vi "begin_conveyor.vi"() -> (0 "error out":errorcluster)   [LabVIEW 2012]
uses:
  <vilib>/Rock Robotics/WPI/CAN/Jaguar/SubVIs/WPI_CANJaguar_BrakeCoastMode.ctl
  <vilib>/Rock Robotics/SystemInterfaces/AI/FPGA_AIChannel.ctl
  <vilib>/Rock Robotics/WPI/MotorControl/WPI_MotorControlOpenCANJaguar.vi
  <vilib>/Rock Robotics/SystemInterfaces/DIO/FPGA_DIOChannel.ctl
  <vilib>/Rock Robotics/SystemInterfaces/Typedef/FPGA_TypedefDigitalModule.ctl
  <vilib>/Rock Robotics/SystemInterfaces/DIO/FPGA_DIOPWMChannel.ctl
  <vilib>/Rock Robotics/WPI/MotorControl/WPI_MotorControlOpen Jaguar.vi
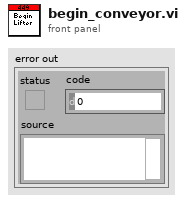
[diagram p1: front panel]
types:
  T1 = typedef "FPGA_AIChannel.ctl" = enum8{"AI 1", "AI 2", "AI 3", "AI 4", "AI 5", "AI 6", "AI 7", "AI 8", "Invalid"}
  T2 = typedef "FPGA_DIOChannel.ctl" = enum8{"DIO 1", "DIO 2", "DIO 3", "DIO 4", "DIO 5", "DIO 6", "DIO 7", "DIO 8", "DIO 9", "DIO 10", "DIO 11", "DIO 12", "DIO 13", "DIO 14", "Invalid"}
  T3 = typedef "WPI_DigitalInputDevRef.ctl" = cluster{"DevStatus":errorcluster, "DIO Channel":T2, "Digital Module":T4}
  T4 = typedef "FPGA_TypedefDigitalModule.ctl" = enum16{"Digital Module 1", "Digital Module 2"}
  T5 = typedef "WPI_CANJaguar_BrakeCoastMode.ctl" = enum8{"Jumper", "Brake", "Coast"}
  T6 = typedef "FPGA_DIOPWMChannel.ctl" = enum8{"PWM 1", "PWM 2", "PWM 3", "PWM 4", "PWM 5", "PWM 6", "PWM 7", "PWM 8", "PWM 9", "PWM 10", "Invalid"}
  T7 = typedef "WPI_MotorControlDeviceRef.ctl" = cluster{"DeviceStatus":errorcluster, "Type":enum16{"PWM", "CAN"}, "PWM":cluster{"Digital Module":T4, "PWM Channel":T6, "DeadBand":T8}, "CAN":cluster{"Device Number":u8, "Control Mode":T9, "Semaphore":T10, "Max Vout":dbl}, "Invert":bool, "TransformRef":T11, "InvTransformRef":T11}
  T8 = typedef "WPI_PWMDeadband.ctl" = cluster{"Name":string, "maxPositivePwm":i32, "minPositivePwm":i32, "centerPwm":i32, "maxNegativePwm":i32, "minNegativePwm":i32, "angularRange":u16}
  T9 = typedef "WPI_CANJaguar_ControlMode.ctl" = enum8{"Percent VBus", "Current", "Speed", "Position", "Voltage"}
  T10 = typedef "Semaphore RefNum" = refnum<k1>
  T11 = typedef "WPI_PWMTransform_ConPane.ctl" = refnum<vi>
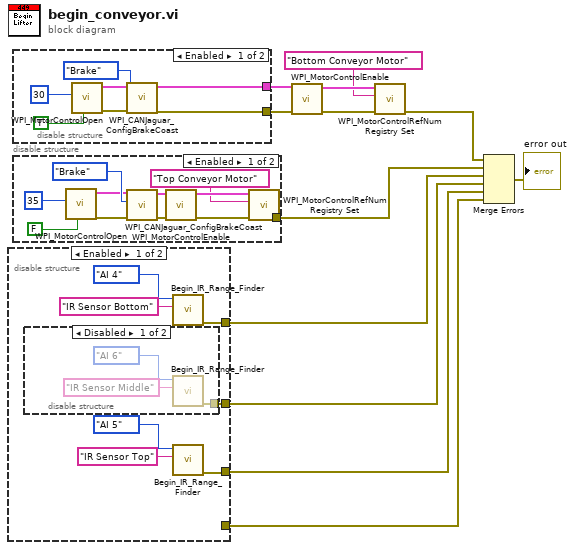
[diagram p0: block diagram]
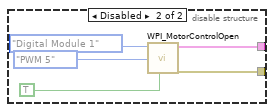
[diagram p2: hidden frame]
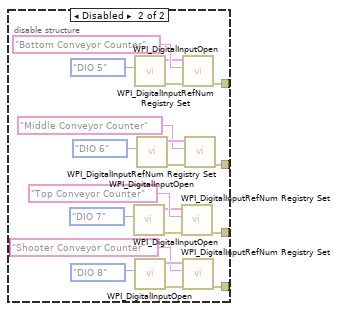
[diagram p5: hidden frame]
diagram:
  n1 = disable-structure shown="Enabled" {
    disable-tunnel: [w17 w39] -> w2
    disable-tunnel: [w16 w25] -> w3
    disable-tunnel: [w13 w24] -> w4
    disable-tunnel: [_ w23] -> w5
    frame Enabled {
      n2 = disable-structure shown="Disabled" {
        disable-tunnel: [w20 _] -> w16
        frame Disabled {
          n3 = call "Begin_IR_Range_Finder.vi"("Reference Name"="IR Sensor Middle", "Analog Channel"=FPGA_AIChannel."AI 6") -> ("error out"=w20:errorcluster)  [unwired: 9 in]
        }
        frame Enabled {
        }
      }
      n4 = call "Begin_IR_Range_Finder.vi"("Reference Name"="IR Sensor Bottom", "Analog Channel"=FPGA_AIChannel."AI 4") -> ("error out"=w17:errorcluster)  [unwired: 9 in]
      n5 = call "Begin_IR_Range_Finder.vi"("Reference Name"="IR Sensor Top", "Analog Channel"=FPGA_AIChannel."AI 5") -> ("error out"=w13:errorcluster)  [unwired: 9 in]
    }
    frame Disabled {
      n6 = call <vilib>:"WPI_DigitalInputOpen.vi"("DIO Channel"=FPGA_DIOChannel."DIO 7") -> ("error out"=w31:errorcluster, "DigitalInputDevRef"=w32:T3)  [unwired: 9 in]
      n7 = call <vilib>:"WPI_DigitalInputOpen.vi"("DIO Channel"=FPGA_DIOChannel."DIO 5") -> ("error out"=w40:errorcluster, "DigitalInputDevRef"=w41:T3)  [unwired: 9 in]
      n8 = call <vilib>:"WPI_DigitalInputOpen.vi"("DIO Channel"=FPGA_DIOChannel."DIO 8") -> ("error out"=w28:errorcluster, "DigitalInputDevRef"=w27:T3)  [unwired: 9 in]
      n9 = call <vilib>:"WPI_DigitalInputOpen.vi"("DIO Channel"=FPGA_DIOChannel."DIO 6") -> ("error out"=w36:errorcluster, "DigitalInputDevRef"=w35:T3)  [unwired: 9 in]
      n10 = call <vilib>:"WPI_DigitalInputRefNum Registry Set.vi"("error in (no error)"=w31, "refnum name"="Top Conveyor Counter", "DigitalInputDevRef"=w32) -> ("error out"=w24:errorcluster)  [unwired: 7 in, 1 out]
      n11 = call <vilib>:"WPI_DigitalInputRefNum Registry Set.vi"("error in (no error)"=w40, "refnum name"="Bottom Conveyor Counter", "DigitalInputDevRef"=w41) -> ("error out"=w39:errorcluster)  [unwired: 7 in, 1 out]
      n12 = call <vilib>:"WPI_DigitalInputRefNum Registry Set.vi"("error in (no error)"=w28, "refnum name"="Shooter Conveyor Counter", "DigitalInputDevRef"=w27) -> ("error out"=w23:errorcluster)  [unwired: 7 in, 1 out]
      n13 = call <vilib>:"WPI_DigitalInputRefNum Registry Set.vi"("error in (no error)"=w36, "refnum name"="Middle Conveyor Counter", "DigitalInputDevRef"=w35) -> ("error out"=w25:errorcluster)  [unwired: 7 in, 1 out]
    }
  }
  n14 = disable-structure shown="Enabled" {
    disable-tunnel: [w47 w54] -> w8
    disable-tunnel: [w46 w50] -> w7
    frame Enabled {
      n15 = call-poly <vilib>:"WPI_MotorControlOpen.vi"("Invert"=TRUE, "Device Number"=u8 30) -> ("error out"=w45:errorcluster, "MotorControlDeviceRef"=w44:T7)  [unwired: 8 in]
      n16 = call <vilib>:"WPI_CANJaguar_ConfigBrakeCoast.vi"("error in (no error)"=w45, "Brake / Coast Mode"=WPI_CANJaguar_BrakeCoastMode."Brake", "CAN Jaguar Ref"=w44) -> ("error out"=w46:errorcluster, "CAN Jaguar Ref Out"=w47:T7)  [unwired: 7 in]
    }
    frame Disabled {
      n17 = call-poly <vilib>:"WPI_MotorControlOpen.vi"("Invert"=TRUE, "PWM Channel"=FPGA_DIOPWMChannel."PWM 5", "Digital Module (Module 1)"=FPGA_TypedefDigitalModule."Digital Module 1") -> ("error out"=w50:errorcluster, "MotorControlDeviceRef"=w54:T7)  [unwired: 7 in]
    }
  }
  n18 = disable-structure shown="Enabled" {
    disable-tunnel: [w55 _] -> w6
    frame Enabled {
      n19 = call-poly <vilib>:"WPI_MotorControlOpen.vi"("Invert"=FALSE, "Device Number"=u8 35) -> ("error out"=w64:errorcluster, "MotorControlDeviceRef"=w63:T7)  [unwired: 8 in]
      n20 = call <vilib>:"WPI_CANJaguar_ConfigBrakeCoast.vi"("error in (no error)"=w64, "Brake / Coast Mode"=WPI_CANJaguar_BrakeCoastMode."Brake", "CAN Jaguar Ref"=w63) -> ("error out"=w61:errorcluster, "CAN Jaguar Ref Out"=w62:T7)  [unwired: 7 in]
      n21 = call <vilib>:"WPI_MotorControlEnable.vi"("error in (no error)"=w61, "CAN Jaguar Ref"=w62) -> ("error out"=w56:errorcluster, "CAN Jaguar Ref Out"=w58:T7)  [unwired: 8 in]
      n22 = call <vilib>:"WPI_MotorControlRefNum Registry Set.vi"("error in (no error)"=w56, "refnum name"="Top Conveyor Motor", "MotorControlDevRef"=w58) -> ("error out"=w55:errorcluster)  [unwired: 7 in, 1 out]
    }
    frame Disabled {
    }
  }
  n23 = call <vilib>:"WPI_MotorControlEnable.vi"("error in (no error)"=w7, "CAN Jaguar Ref"=w8) -> ("error out"=w11:errorcluster, "CAN Jaguar Ref Out"=w12:T7)  [unwired: 8 in]
  n24 = call <vilib>:"WPI_MotorControlRefNum Registry Set.vi"("error in (no error)"=w11, "refnum name"="Bottom Conveyor Motor", "MotorControlDevRef"=w12) -> ("error out"=w9:errorcluster)  [unwired: 7 in, 1 out]
  n25 = Merge Errors(w9, w6, w2, w3, w4, w5) -> (→"error out":errorcluster)
